vi "ACQUISITION_Echo.vi"() -> ()   [LabVIEW 2025]
uses:
  <vilib>/express/express analysis/Spectral/Block/exnSpectralBlock spectral measurements RMS poly.vi
  <vilib>/express/express analysis/Spectral/Block/exnSpectralBlock spectral measurements RMS DDT.vi
  <vilib>/express/express analysis/Spectral/XNode/ExpressSpectralMeasurementsBlockNode.xnode
panel:
  out "FFT du signal":dynamicdata(graph)
  out "Signal après fenêtrage":dynamicdata(graph)
  out "Signal Différenciel sur AI0":dynamicdata(graph)
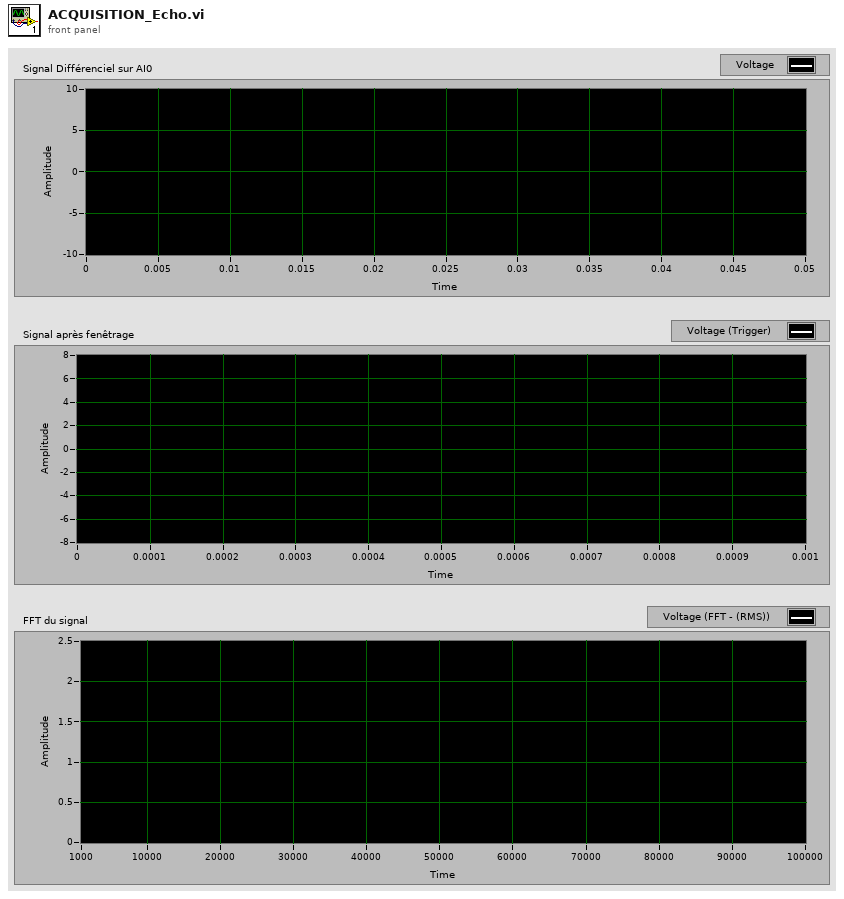
[diagram p1: front panel]
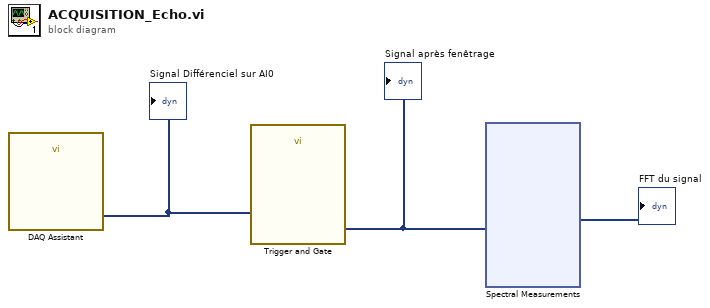
[diagram p0: block diagram]
diagram:
  n1 = call "DAQ Assistant"() -> ("data"=w3:dynamicdata)  [unwired: 17 in, 2 out]
  "Signal Différenciel sur AI0" <- w3
  n2 = call "Trigger and Gate"("Signals"=w3) -> ("Triggered Signals"=w1:dynamicdata)  [unwired: 7 in, 3 out]
  "Signal après fenêtrage" <- w1
  n3 = xnode "Spectral Measurements"("Signals"=w1) -> ("FFT - (RMS)"=→"FFT du signal":dynamicdata)  [unwired: 2 in, 3 out]
